vi "DCA Calibration INI File.vi"(8 "error in (no error)":errorcluster, 10 "Operation":enum16{"Read", "Write", "Clear"}(ring), 11 "Calibration In":T1) -> (0 "error out":errorcluster, 3 "Calibration Out":T1)   [LabVIEW 2011]
uses:
  TypeDefs/DCA Calibration State.ctl
  <vilib>/Utility/config.llb/Read Key (String).vi
  <vilib>/Utility/config.llb/Write Key (String).vi
  <vilib>/Utility/config.llb/NI_LVConfig.lvlib
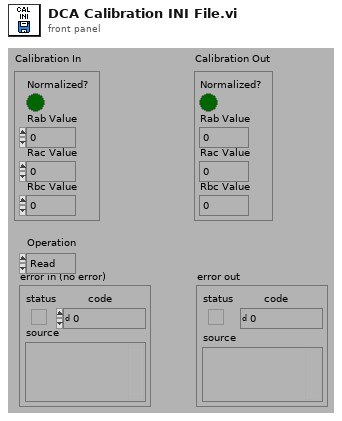
[diagram p1: front panel]
types:
  T1 = typedef "DCA Calibration State.ctl" = cluster{"Normalized?":bool, "Rab Value":dbl, "Rac Value":dbl, "Rbc Value":dbl}
  T2 = typedef "NI_LVConfig.lvlib/Config Data RefNum.ctl" = refnum<k1>
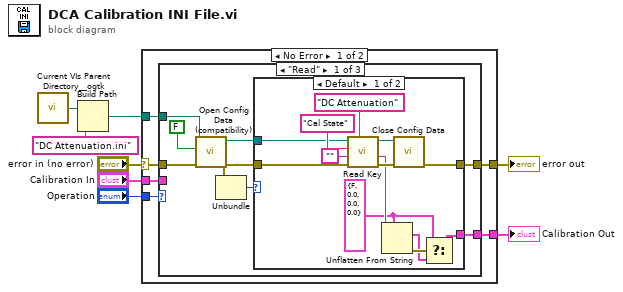
[diagram p0: block diagram]
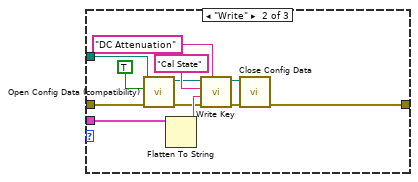
[diagram p3: hidden frame]
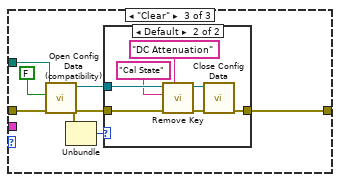
[diagram p4: hidden frame]
diagram:
  n1 = call "Current VIs Parent Directory__ogtk.vi"() -> ("Parent Directory (+ Relative)"=w1:path)  [unwired: 5 in]
  n2 = Build Path(base path=w1, name or relative path="DC Attenuation.ini") -> (appended path=w7:path)
  n3 = case shown="No Error" "error in (no error)" {
    selector: "error in (no error)" -> [w9 w62]
    tunnel: w7 -> [w14 _]
    tunnel: [w13 w62] -> w6
    tunnel: [w12 _] -> w5
    tunnel: "Operation" -> [w11 _]
    tunnel: "Calibration In" -> [w10 _]
    frame No Error {
      n4 = case shown="\"Read\"" w11 {
        tunnel: w14 -> [w19 w38 w50]
        tunnel: w9 -> [w18 w39 w49]
        tunnel: [w22 w37 w48] -> w13
        tunnel: [w21 _ _] -> w12
        tunnel: w10 -> [_ w36 _]
        frame "Read" {
          n5 = call <vilib>:"Open Config Data (compatibility).vi"("error in (no error)"=w18, "create file if necessary (T)"=FALSE ("create file if necessary? (T)"), "configuration file path"=w19) -> ("error out"=w17:errorcluster, "refnum"=w20:T2)  [unwired: 6 in, 1 out]
          n6 = Unbundle(w17) -> ("code"=w16:i32)  [unwired: 2 out]
          n7 = case shown="Default" w16 {
            tunnel: w17 -> [w28 _]
            tunnel: [w35 _] -> w22
            tunnel: w20 -> [w27 _]
            tunnel: [w24 _] -> w21
            frame Default {
              w23 = T1 {"Normalized?"=FALSE, "Rab Value"=0.0, "Rac Value"=0.0, "Rbc Value"=0.0} ("Calibration")
              n8 = call-poly <vilib>:"Read Key.vi"("section"="DC Attenuation" ("name or relative path"), "error in (no error)"=w28, "default value"="", "key"="Cal State" ("format string"), "refnum"=w27) -> ("error out"=w32:errorcluster, "value"=w30:string, "refnum out"=w33:T2)  [unwired: 1 in, 3 out]
              n9 = Unflatten From String(type=w23, binary string=w30) -> (value=w25:T1, error out=w26:errorcluster)  [unwired: 1 in, 3 out]
              n10 = call <vilib>:"Close Config Data.vi"("error in (no error)"=w32, "refnum"=w33) -> ("error out"=w35:errorcluster)  [unwired: 1 in, 8 out]
              n11 = Select(t=w23, s=w26, f=w25) -> (s? t:f=w24:T1)
            }
            frame 7 {
            }
          }
        }
        frame "Write" {
          n12 = call <vilib>:"Open Config Data (compatibility).vi"("error in (no error)"=w39, "create file if necessary (T)"=TRUE ("create file if necessary? (T)"), "configuration file path"=w38) -> ("error out"=w41:errorcluster, "refnum"=w42:T2)  [unwired: 6 in, 1 out]
          n13 = Flatten To String(anything=w36) -> (data string=w46:string)  [unwired: 1 in, 4 out]
          n14 = call-poly <vilib>:"Write Key.vi"("section"="DC Attenuation", "error in (no error)"=w41, "value"=w46, "key"="Cal State" ("format string"), "refnum"=w42) -> ("error out"=w44:errorcluster, "refnum out"=w45:T2)  [unwired: 1 in, 4 out]
          n15 = call <vilib>:"Close Config Data.vi"("error in (no error)"=w44, "refnum"=w45) -> ("error out"=w37:errorcluster)  [unwired: 1 in, 8 out]
        }
        frame "Clear" {
          n16 = call <vilib>:"Open Config Data (compatibility).vi"("error in (no error)"=w49, "create file if necessary (T)"=FALSE ("create file if necessary? (T)"), "configuration file path"=w50) -> ("error out"=w52:errorcluster, "refnum"=w54:T2)  [unwired: 6 in, 1 out]
          n17 = Unbundle(w52) -> ("code"=w51:i32)  [unwired: 2 out]
          n18 = case shown="Default" w51 {
            tunnel: w52 -> [_ w61]
            tunnel: w54 -> [_ w60]
            tunnel: [_ w59] -> w48
            frame 7 {
            }
            frame Default {
              n19 = call <vilib>:"Remove Key.vi"("section"="DC Attenuation" ("name or relative path"), "error in (no error)"=w61, "key"="Cal State" ("name or relative path"), "refnum"=w60) -> ("error out"=w56:errorcluster, "refnum out"=w55:T2)  [unwired: 6 out]
              n20 = call <vilib>:"Close Config Data.vi"("error in (no error)"=w56, "refnum"=w55) -> ("error out"=w59:errorcluster)  [unwired: 1 in, 8 out]
            }
          }
        }
      }
    }
    frame Error {
    }
  }
  "error out" <- w6
  "Calibration Out" <- w5
